vi "InterpolateTemperatureVoltagePairs.vi"(7 "Configuration":T1, 8 "error in":errorcluster, 9 "V & T Pairs":i32, 10 "Average Temperatures (Cº)":dbl[](array[numeric]), 11 "Average Voltages":dbl[][](array[numeric])) -> (0 "error out":errorcluster, 1 "Fit Errors":dbl[](array[numeric]), 2 "Fit Coefficients":dbl[][](array[numeric]), 5 "TvsR_Array":cluster{"Temperatures":dbl[], dbl[]}[](array[cluster]))   [LabVIEW 2014]
uses:
  Settings/Settings.ctl
  Acquisition/Hardware Configuration.ctl
  Logging/Logging Configuration.ctl
  <vilib>/Analysis/NI_AALPro.lvlib
  Acquisition/Acquisition.lvlib
  Settings/Settings.lvlib
  Logging/Logging.lvlib
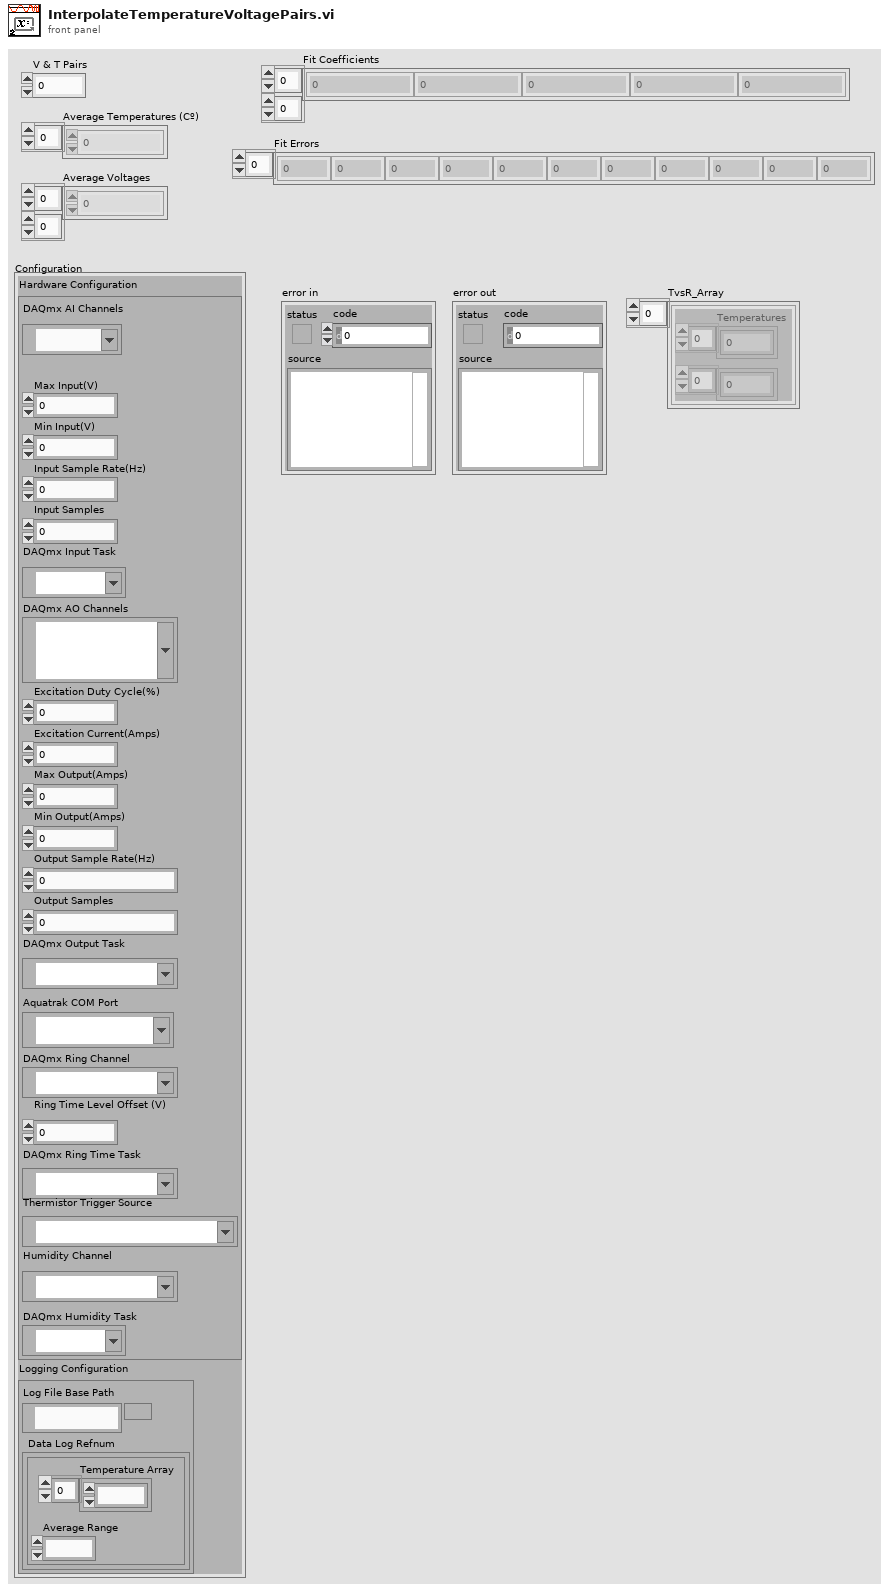
[diagram p1: front panel]
types:
  T1 = typedef "Settings.lvlib/Settings.ctl" = cluster{"Hardware Configuration":T2, "Logging Configuration":T3}
  T2 = typedef "Acquisition.lvlib/Hardware Configuration.ctl" = cluster{"DAQmx AI Channels":tag, "Max Input(V)":dbl, "Min Input(V)":dbl, "Input Sample Rate(Hz)":dbl, "Input Samples":dbl, "DAQmx Input Task":refnum<k21>, "DAQmx AO Channels":tag, "Excitation Duty Cycle(%)":dbl, "Excitation Current(Amps)":dbl, "Max Output(Amps)":dbl, "Min Output(Amps)":dbl, "Output Sample Rate(Hz)":dbl, "Output Samples":dbl, "DAQmx Output Task":refnum<k21>, "Aquatrak COM Port":refnum<visa-resource-name>, "DAQmx Ring Channel":tag, "Ring Time Level Offset (V)":dbl, "DAQmx Ring Time Task":refnum<k21>, "Thermistor Trigger Source":tag, "Humidity Channel":tag, "DAQmx Humidity Task":refnum<k21>}
  T3 = typedef "Logging.lvlib/Logging Configuration.ctl" = cluster{"Log File Base Path":path, "Data Log Refnum":refnum<k1>}
  T4 = cluster{"Average Temperatures (Cº)":dbl[], dbl[]}
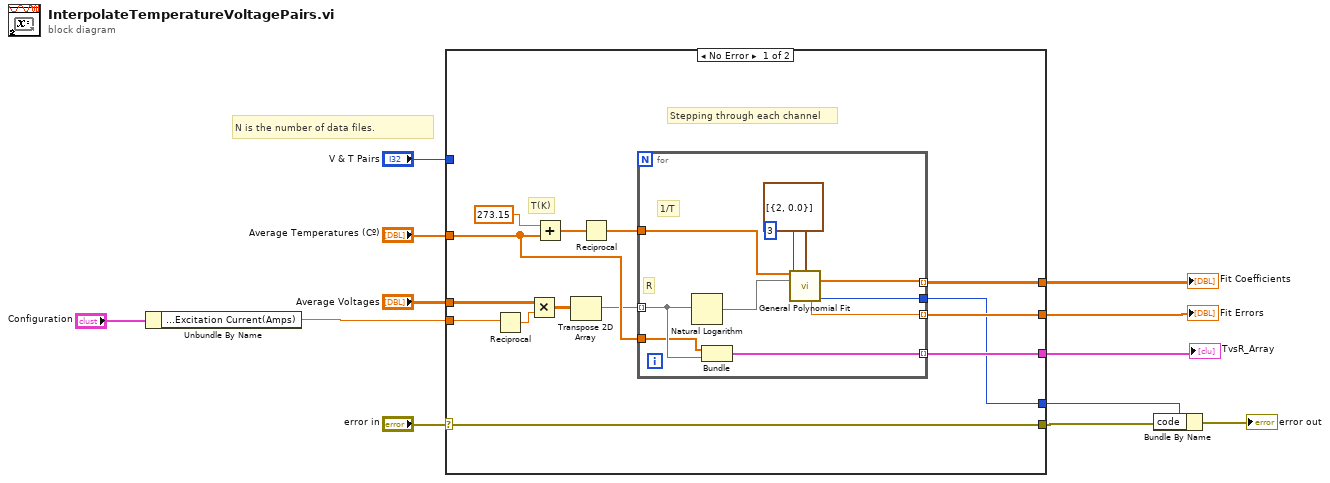
[diagram p0: block diagram]
diagram:
  # "N is the number of data files."
  n1 = Unbundle By Name("Configuration") -> ("Hardware Configuration.Excitation Current(Amps)"=w7:dbl)
  n2 = case shown="No Error" "error in" {
    selector: "error in" -> [w13 w37]
    tunnel: "Average Temperatures (Cº)" -> [w26 _]
    tunnel: "Average Voltages" -> [w23 _]
    tunnel: "V & T Pairs" -> [_ _]
    tunnel: [w13 w37] -> w2
    tunnel: w7 -> [w25 _]
    tunnel: [w17 _] -> w6
    tunnel: [w16 _] -> w5
    tunnel: [w15 _] -> w4
    tunnel: [w14 _] -> w3
    frame No Error {
      # "T(K)"
      # "Stepping through each channel"
      n3 = Reciprocal(x=w25) -> (1/x=w24:dbl)
      n4 = Multiply(x=w23, y=w24) -> (x*y=w22:dbl[][])
      n5 = Add(x=273.15, y=w26) -> (x+y=w20:dbl[])
      n6 = Transpose 2D Array(2D array=w22) -> (transposed array=w18:dbl[][])
      n7 = Reciprocal(x=w20) -> (1/x=w19:dbl[])
      n8 = for {
        tunnel: w18 -> [w30] mode=indexing
        tunnel: w19 -> [w33]
        tunnel: [w36] -> w17 mode=indexing
        tunnel: [w31] -> w14
        tunnel: w26 -> [w29]
        tunnel: [w28] -> w15 mode=indexing
        tunnel: [w27] -> w16 mode=indexing
        # "1/T"
        # "R"
        n9 = Natural Logarithm(1:w30) -> (0:w32:dbl[])
        n10 = Bundle("Average Temperatures (Cº)"=w29, w30) -> (w28:T4)  [unwired: 1 in]
        n11 = call <vilib>:"General Polynomial Fit.vi"("Y"=w33, "polynomial order"=3, "Coefficient Constraint"=cluster{"order":i32, "coefficient":dbl}[] [{"order"=2, "coefficient"=0.0}], "X"=w32) -> ("Polynomial Coefficients"=w36:dbl[], "residue"=w27:dbl, "error"=w31:i32)  [unwired: 8 in, 1 out]
      }
    }
    frame Error {
    }
  }
  "Fit Coefficients" <- w6
  "TvsR_Array" <- w4
  "Fit Errors" <- w5
  n12 = Bundle By Name(cluster=w2, "code"=w3) -> (→"error out":errorcluster)
